vi "비전샘플.vi"() -> ()   [LabVIEW 2020]
uses:
  <vilib>/vision/Pattern Matching.llb/IMAQ Curve Parameters.ctl
  <vilib>/vision/NI_Vision_Development_Module.lvlib
panel:
  in  "템플릿 저장 경로":path
  in  "정지":bool
  in  "템플릿 생성":bool
  in  "판별":bool
  out "템플릿":T1(plugin-control)
  out "Image":T1(plugin-control)
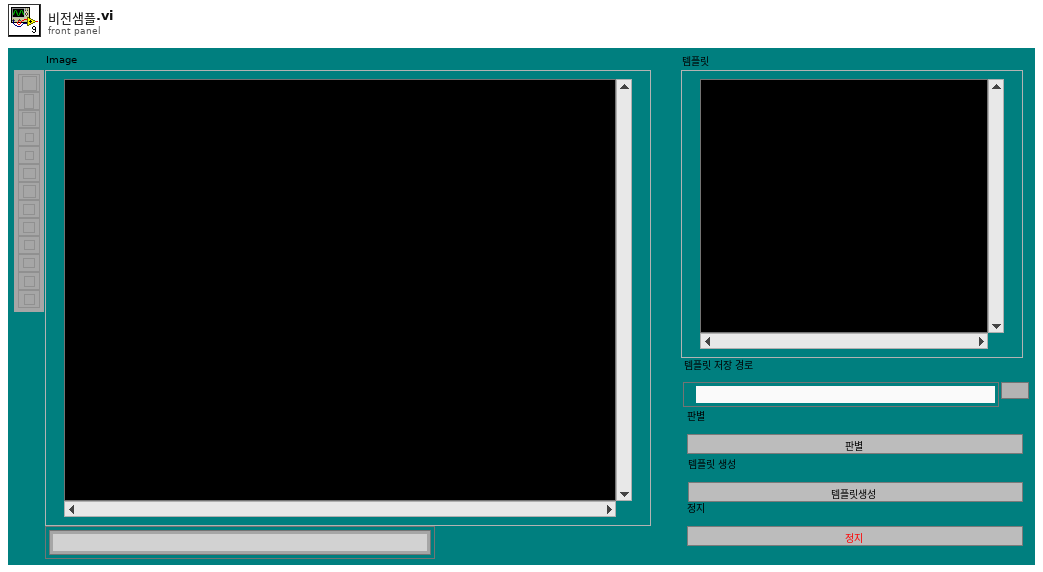
[diagram p1: front panel]
types:
  T1 = typedef "IMAQ Image.ctl" = refnum<image>
  T2 = typedef "Image Type" = u32
  T3 = typedef "IMAQ Curve Parameters.ctl" = cluster{"Extraction Mode":u32, "Edge Threshold":i32, "Edge Filter Size":u32, "Min Length":i32, "Row Search Step Size":i32, "Col Search Step Size":i32, "Max Endpoint Gap":i32, "Closed":bool, "Subpixel":bool}
  T4 = typedef "ROI Descriptor" = cluster{"Global Rectangle":i32[], "Contours":cluster{"ID":enum32{"External", "Internal"}, "Type":u32, "Coordinates":i32[]}[]}
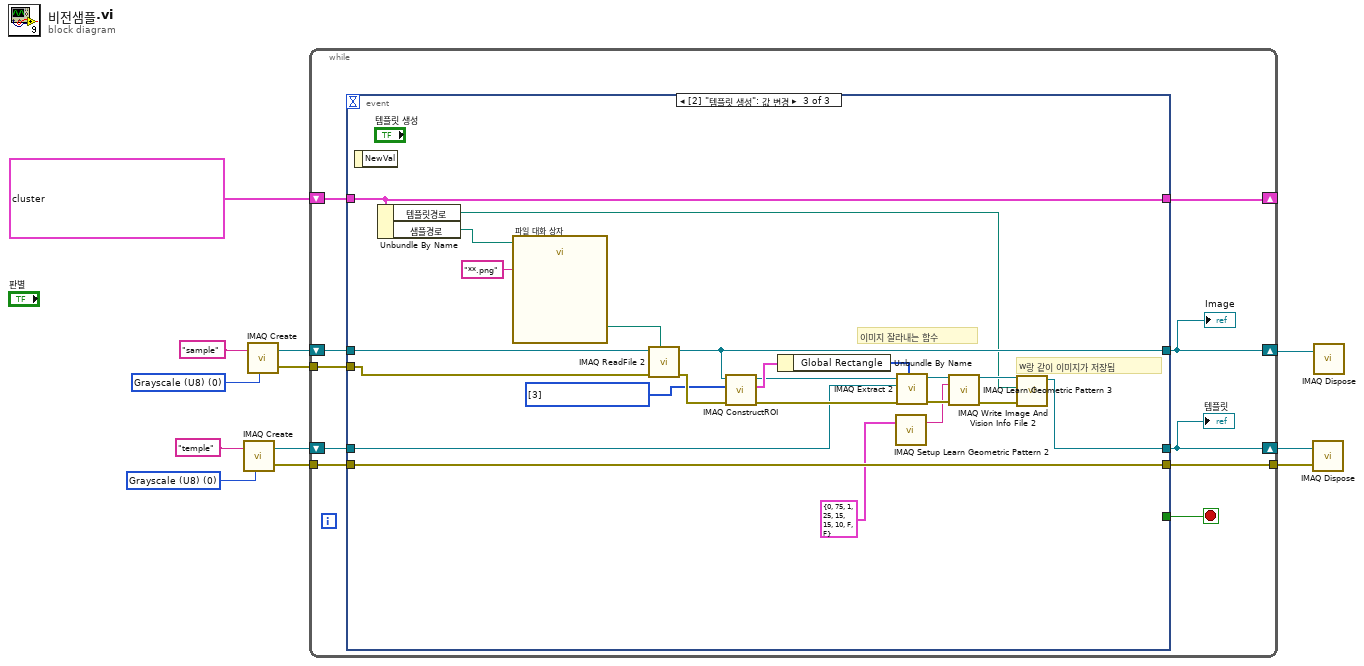
[diagram p0: block diagram]
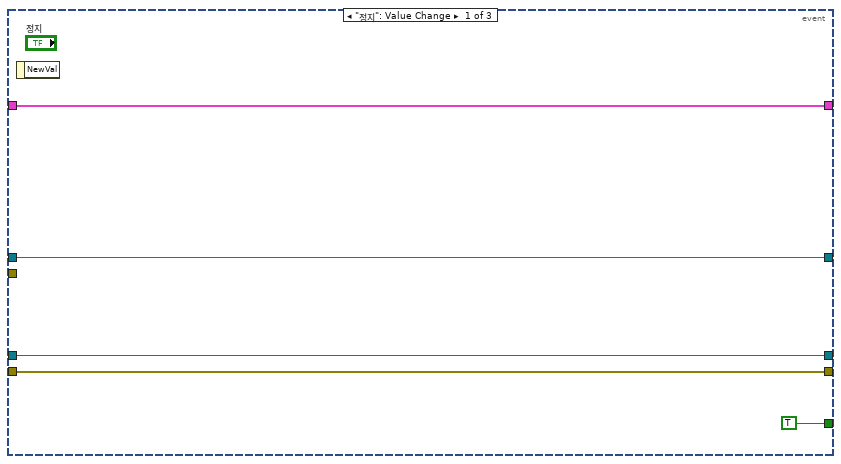
[diagram p2: hidden frame]
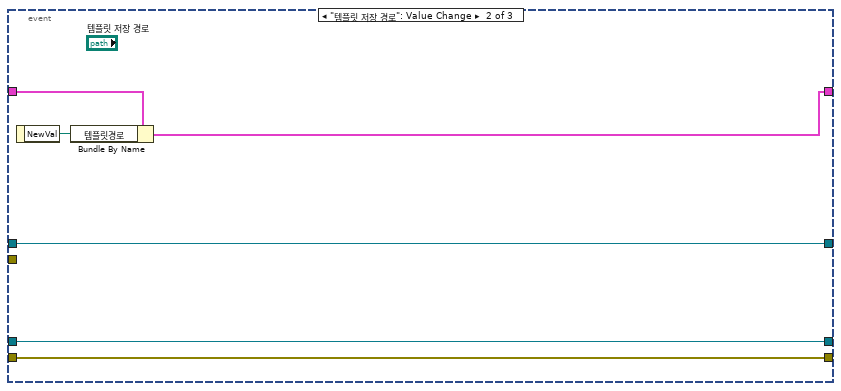
[diagram p3: hidden frame]
diagram:
  w9 = T2 0 items=["Grayscale (U8)", "Grayscale (I16)", "Grayscale (SGL)", "Complex (CSG)", "RGB (U32)", "HSL (U32)", "RGB (U64)", "Grayscale (U16)"] ("Image Type")
  w10 = T2 0 items=["Grayscale (U8)", "Grayscale (I16)", "Grayscale (SGL)", "Complex (CSG)", "RGB (U32)", "HSL (U32)", "RGB (U64)", "Grayscale (U16)"] ("Image Type")
  n1 = call "IMAQ Create"("Image Name"="temple", "Image Type"=w9) -> ("New Image"=w4:T1, "error out"=w5:errorcluster)  [unwired: 3 in]
  n2 = call "IMAQ Create"("Image Name"="sample", "Image Type"=w10) -> ("New Image"=w6:T1, "error out"=w7:errorcluster)  [unwired: 3 in]
  n3 = while {
    shift-right: [w21] -> _
    shift-left: cluster{"샘플경로":path, "템플릿경로":path} {"샘플경로"=path "C:/Users/user/Desktop/일일노트/1007/이미지파일/Parts", "템플릿경로"=path "C:/Users/user/Desktop/일일노트/1007/이미지파일/Parts/템플릿.png"} -> [w22]
    tunnel: w7 -> [w19]
    tunnel: w5 -> [w17]
    shift-right: [w15] -> w3
    shift-left: w6 -> [w18]
    shift-right: [w14] -> w2
    shift-left: w4 -> [w16]
    tunnel: [w13] -> w1
    stop <- w20 stop-if-true
    n4 = event shown="[2] \"템플릿 생성\": 값 변경" {
      selector: _ -> [_ _ _]
      dyn-events: _ -> [_ _ _]
      timeout: _ -> [_ _ _]
      tunnel: w22 -> [w27 w30 w55]
      tunnel: [w27 w28 w55] -> w21
      tunnel: [TRUE _ _] -> w20
      tunnel: w19 -> [_ _ w50]
      tunnel: w18 -> [w25 w33 w52]
      tunnel: w17 -> [w23 w31 w56]
      tunnel: w16 -> [w24 w32 w35]
      tunnel: [w25 w33 w43] -> w15
      tunnel: [w24 w32 w36] -> w14
      tunnel: [w23 w31 w56] -> w13
      event "정지": Value Change {
        n5 = event-data() -> ()  [unwired: 1 in, 1 out]
      }
      event "템플릿 저장 경로": Value Change {
        n6 = event-data() -> ("NewVal"=w29:path)  [unwired: 1 in]
        n7 = Bundle By Name(cluster=w30, "템플릿경로"=w29) -> (w28:cluster{"샘플경로":path, "템플릿경로":path})
      }
      event "템플릿 생성": Value Change {
        w48 = u32[] [3] items=["No Selection", "Point", "Line", "Rectangle", "Oval", "Polygon", "Freehand Region", "Annulus", "Zoom", "Pan", "Broken Line", "Freehand Line", "Rotated Rectangle"] ("Tools")
        # "w랑 같이 이미지가 저장됨"
        # "이미지 잘라내는 함수"
        n8 = event-data() -> ()  [unwired: 1 in, 1 out]
        n9 = Unbundle By Name(w55) -> ("템플릿경로"=w34:path, "샘플경로"=w54:path)
        n10 = call "파일 대화 상자"("start path"=w54, "pattern (all files)"="**.png") -> ("selected path"=w51:path)  [unwired: 10 in, 3 out]
        n11 = call "IMAQ ReadFile 2"("File Path"=w51, "error in (no error)"=w50, "Image"=w52) -> ("error out"=w49:errorcluster, "Image Out"=w43:T1)  [unwired: 4 in, 3 out]
        n12 = call "IMAQ ConstructROI"("error in (no error)"=w49, "Tools"=w48, "Image"=w43) -> ("error out"=w44:errorcluster, "ROI Descriptor Out"=w47:T4, "Image Out (duplicate)"=w45:T1)  [unwired: 5 in, 1 out]
        n13 = Unbundle By Name(w47) -> ("Global Rectangle"=w46:i32[])
        n14 = call "IMAQ Setup Learn Geometric Pattern 2"("Curve Parameters"=T3 {"Extraction Mode"=0, "Edge Threshold"=75, "Edge Filter Size"=1, "Min Length"=25, "Row Search Step Size"=15, "Col Search Step Size"=15, "Max Endpoint Gap"=10, "Closed"=FALSE, "Subpixel"=FALSE}) -> ("Learn Geometric Pattern 2 Setup Data"=w40:string)  [unwired: 1 in, 1 out]
        n15 = call "IMAQ Extract 2"("Optional Rectangle"=w46, "error in (no error)"=w44, "Image Dst"=w35, "Image Src"=w45) -> ("error out"=w41:errorcluster, "Image Dst Out"=w42:T1)  [unwired: 6 in]
        n16 = call "IMAQ Learn Geometric Pattern 3"("Template Image"=w42, "Learn Geometric Pattern 2 Setup Data"=w40, "error in (no error)"=w41) -> ("Template Image Out"=w38:T1, "error out"=w37:errorcluster)  [unwired: 11 in]
        n17 = call "IMAQ Write Image And Vision Info File 2"("error in (no error)"=w37, "File Path"=w34, "Image"=w38) -> ("Image Out (duplicate)"=w36:T1)  [unwired: 7 in, 1 out]
      }
    }
    "Image" <- w15
    "템플릿" <- w14
  }
  n18 = call "IMAQ Dispose"("Image"=w2, "error in (no error)"=w1) -> ()  [unwired: 4 in, 1 out]
  n19 = call "IMAQ Dispose"("Image"=w3) -> ()  [unwired: 5 in, 1 out]
